vi "GetSponsorLogos.vi"(7 "LabVIEW Web Service Request":refnum<class "Web Request.lvclass">) -> ()   [LabVIEW 2013]
uses:
  <vilib>/wsapi/Web Request.lvclass
panel:
  # "Use the Web Service Request input terminal to call the VIs on the Web Services palette. Do not remove it from the connector pane unless you don't need access to the palette."
  # "Each additional control wired to the connector pane will be available as an input in the URL. To include an indicator in terminal-mode output (the default setting), it must also be wired to the connector pane."
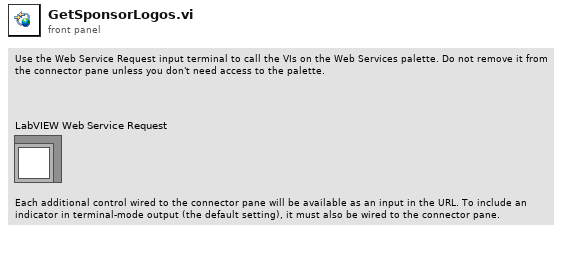
[diagram p1: front panel]
types:
  T1 = typedef "ImageInfoList.ctl" = cluster{"Image Array":cluster{"Alias":string, "Path":path}[], "Frequency (s)":dbl}
  T2 = typedef "imagedata.ctl" = cluster{"image type":i32, "image depth":i32, "image":u8[], "mask":u8[], "colors":u32[], "Rectangle":cluster{"left":i16, "top":i16, "right":i16, "bottom":i16}}
  T3 = cluster{"Cluster":cluster{T2[], "Frequency (s)":dbl}, "Cluster":cluster{T2[], "Frequency (s)":dbl}, "Cluster":cluster{T2[], "Frequency (s)":dbl}}
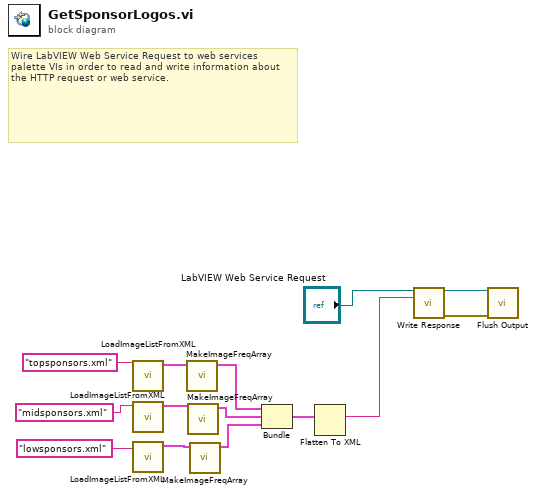
[diagram p0: block diagram]
diagram:
  # "Wire LabVIEW Web Service Request to web services palette VIs in order to read and write information about the HTTP request or web service."
  n1 = call "LoadImageListFromXML.vi"("filename"="topsponsors.xml") -> ("Top Sponsor Image List"=w11:T1)  [unwired: 10 in]
  n2 = call "LoadImageListFromXML.vi"("filename"="midsponsors.xml") -> ("Top Sponsor Image List"=w10:T1)  [unwired: 10 in]
  n3 = call "LoadImageListFromXML.vi"("filename"="lowsponsors.xml") -> ("Top Sponsor Image List"=w9:T1)  [unwired: 10 in]
  n4 = call "MakeImageFreqArray.vi"("Top Sponsor Image List"=w11) -> ("Cluster"=w8:cluster{T2[], "Frequency (s)":dbl})  [unwired: 10 in]
  n5 = call "MakeImageFreqArray.vi"("Top Sponsor Image List"=w10) -> ("Cluster"=w7:cluster{T2[], "Frequency (s)":dbl})  [unwired: 10 in]
  n6 = call "MakeImageFreqArray.vi"("Top Sponsor Image List"=w9) -> ("Cluster"=w6:cluster{T2[], "Frequency (s)":dbl})  [unwired: 10 in]
  n7 = Bundle("Cluster"=w8, "Cluster"=w7, "Cluster"=w6) -> (w5:T3)  [unwired: 1 in]
  n8 = Flatten To XML(anything=w5) -> (xml string=w1:string)
  n9 = call <vilib>:"Write Response.vi"("LabVIEW Web Service Request"="LabVIEW Web Service Request", "response string"=w1) -> ("LabVIEW Web Service Request out"=w3:refnum<class "Web Request.lvclass">, "error out"=w4:errorcluster)  [unwired: 12 in]
  n10 = call <vilib>:"Flush Output.vi"("LabVIEW Web Service Request"=w3, "error in (no error)"=w4) -> ()  [unwired: 12 in, 2 out]
